vi "Problem1.11.vi"() -> ()   [LabVIEW 2019]
panel:
  out "millisecond timer value 2":u32
  out "millisecond timer value":u32
  out "Problem 1.9 Execution Time":u32
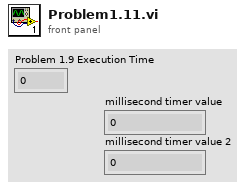
[diagram p1: front panel]
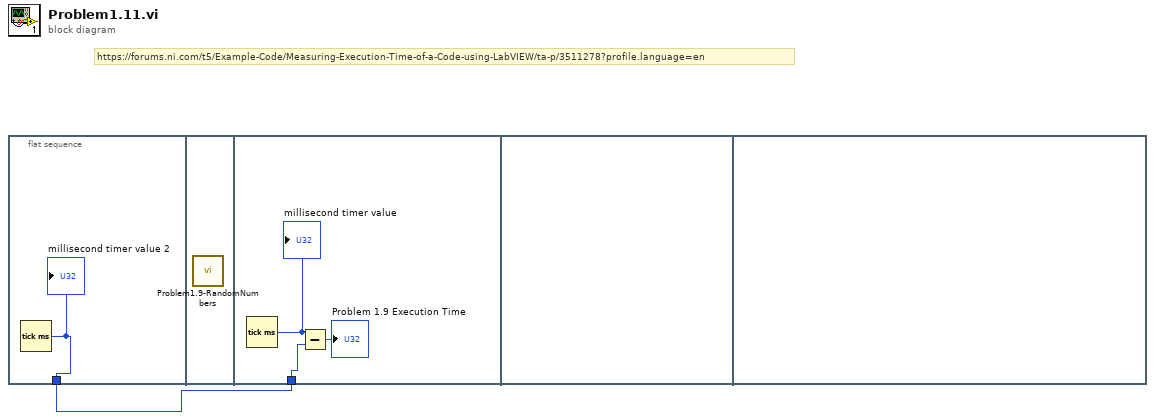
[diagram p0: block diagram]
diagram:
  # "https://forums.ni.com/t5/Example-Code/Measuring-Execution-Time-of-a-Code-using-LabVIEW/ta-p/3511278?profile.language=en"
  n1 = flat-sequence {
    tunnel: [w2] -> w1
    tunnel: w1 -> [w4]
    frame #0 {
      n2 = Tick Count (ms)() -> (millisecond timer value=w2:u32)
      "millisecond timer value 2" <- w2
    }
    frame #1 {
      n3 = call "Problem1.9-RandomNumbers.vi"() -> ()  [unwired: 12 in]
    }
    frame #2 {
      n4 = Tick Count (ms)() -> (millisecond timer value=w5:u32)
      "millisecond timer value" <- w5
      n5 = Subtract(x=w5, y=w4) -> (x-y=→"Problem 1.9 Execution Time":u32)
    }
    frame #3 {
    }
    frame #4 {
    }
  }
